vi "Loop Complete Message.vi"(7 "QRD":T1, 8 "error in":errorcluster, 11 "Loop ID":string) -> (0 "error out":errorcluster, 3 "Loop ID Out":string, 5 "QRD Out":T1)   [LabVIEW 2025]
uses:
  Controls/Queues-Refs-Data.ctl
  Builds/Queue Wrappers.lvlibp/Q Packet.ctl
  Builds/Queue Wrappers.lvlibp
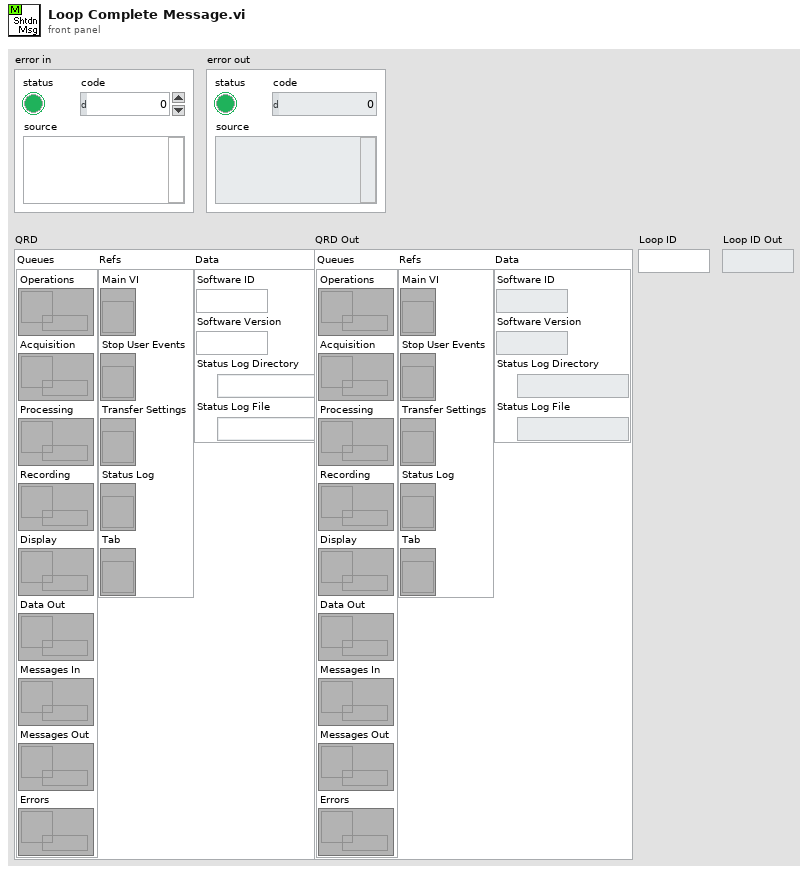
[diagram p1: front panel]
types:
  T1 = typedef "Queues-Refs-Data.ctl" = cluster{"Queues":cluster{"Operations":refnum<queue>, "Acquisition":refnum<queue>, "Processing":refnum<queue>, "Recording":refnum<queue>, "Display":refnum<queue>, "Data Out":refnum<queue>, "Messages In":refnum<queue>, "Messages Out":refnum<queue>, "Errors":refnum<queue>}, "Refs":cluster{"Main VI":refnum<vi>, "Stop User Events":refnum<vi>, "Transfer Settings":refnum<vi>, "Status Log":refnum<vi>, "Tab":refnum<vi>}, "Data":cluster{"Software ID":string, "Software Version":string, "Status Log Directory":path, "Status Log File":path}}
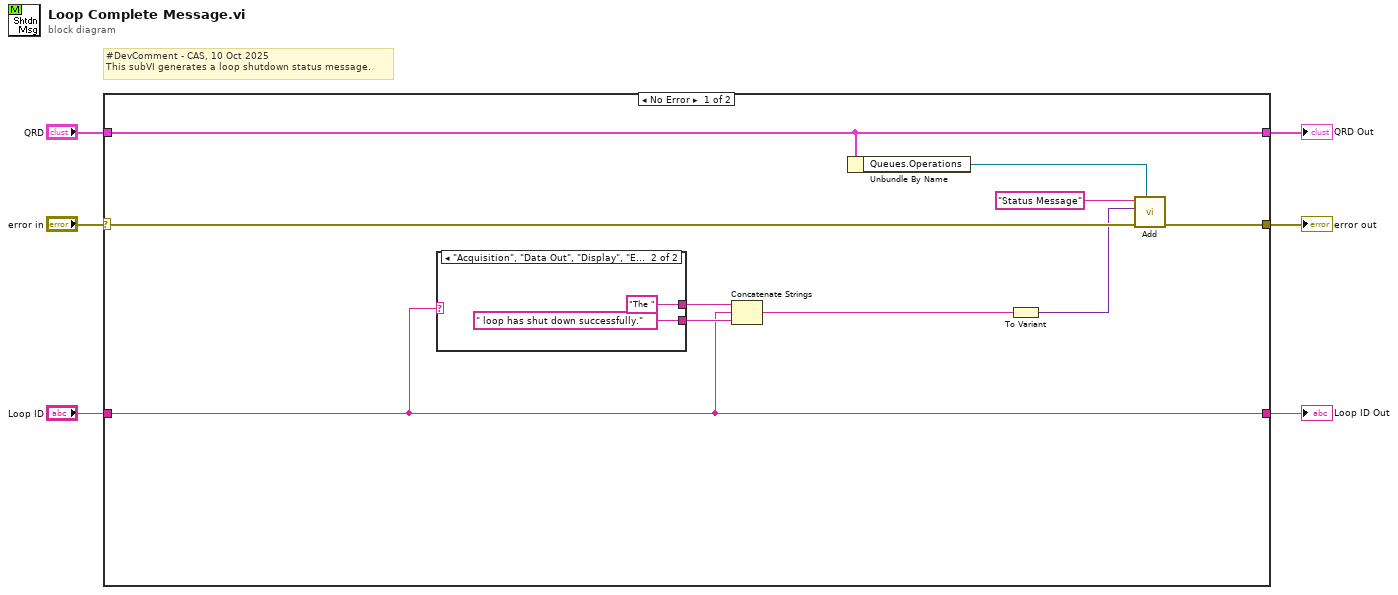
[diagram p0: block diagram]
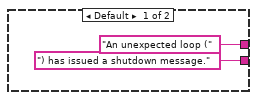
[diagram p2: hidden frame]
diagram:
  # "#DevComment - CAS, 10 Oct 2025\nThis subVI generates a loop shutdown status message."
  n1 = case shown="No Error" "error in" {
    selector: "error in" -> [w16 w21]
    tunnel: "QRD" -> [w12 w23]
    tunnel: [w12 w23] -> w4
    tunnel: [w11 w21] -> w3
    tunnel: "Loop ID" -> [w7 w22]
    tunnel: [w7 w22] -> w1
    frame No Error {
      n2 = case shown="\"Acquisition\", \"Data Out\", \"Display\", \"Errors\", \"Messages In\", \"Messages Out\", \"Processing\", \"Recording\", \"User Events\"" w7 {
        tunnel: ["An unexpected loop (" "The " ("string")] -> w10
        tunnel: [") has issued a shutdown message." " loop has shut down successfully." ("string")] -> w9
        frame Default {
        }
        frame "Acquisition", "Data Out", "Display", "Errors", "Messages In", "Messages Out", "Processing", "Recording", "User Events" {
        }
      }
      n3 = Concatenate Strings(w10, w7, w9) -> (w8:string)
      n4 = Unbundle By Name(w12) -> ("Queues.Operations"=w13:refnum<queue>)
      n5 = To Variant(anything=w8) -> (Variant=w15:variant)
      n6 = call "Add.vi"("Q Ref In"=w13, "error in"=w16, "Payload"=w15, "Packet ID"="Status Message") -> ("error out"=w11:errorcluster)  [unwired: 4 in, 3 out]
    }
    frame Error {
    }
  }
  "error out" <- w3
  "QRD Out" <- w4
  "Loop ID Out" <- w1
